vi "ReadAndConvertFile.vi"(8 "error in (no error)":errorcluster, 10 "Path":path, 11 "GXML in":refnum<class "GXML.lvclass">) -> (0 "error out":errorcluster, 2 "EPT Pattern":T1, 3 "GXML out":refnum<class "GXML.lvclass">)   [LabVIEW 2017, in "File Formats.lvlib" / "GXML.lvclass"]
uses:
  GXML.lvclass
  Parent/EST Pattern.ctl
  <vilib>/NI/GXML/_subVIs/GXML Quick Parser/Quick Parser.vi
  <vilib>/NI/GXML/GXML.lvlib
  Parent/FileFormat.lvclass
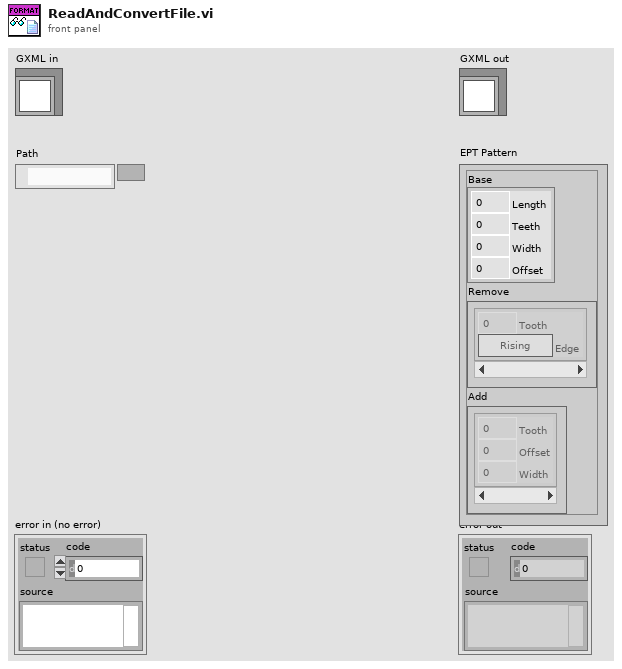
[diagram p1: front panel]
types:
  T1 = typedef "File Formats.lvlib/FileFormat.lvclass/EST Pattern.ctl" = cluster{"Base":cluster{"Length":dbl, "Teeth":u16, "Width":dbl, "Offset":dbl}, "Remove":cluster{"Tooth":u16, "Edge":bool}[], "Add":cluster{"Tooth":u16, "Offset":dbl, "Width":dbl}[]}
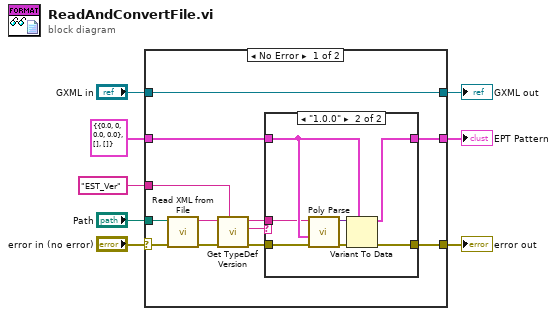
[diagram p0: block diagram]
diagram:
  n1 = case shown="No Error" "error in (no error)" {
    selector: "error in (no error)" -> [w11 w32]
    tunnel: [w12 w32] -> w8
    tunnel: [w20 w31] -> w2
    tunnel: "GXML in" -> [w20 w31]
    tunnel: "EST_Ver" -> [w14 _]
    tunnel: [w13 w30] -> w7
    tunnel: T1 {"Base"={"Length"=0.0, "Teeth"=0, "Width"=0.0, "Offset"=0.0}, "Remove"=[], "Add"=[]} ("EPT Pattern") -> [w10 w30]
    tunnel: "Path" -> [w9 _]
    frame No Error {
      n2 = call <vilib>:"Read XML from File.vi"("error in"=w11, "XML File Path"=w9) -> ("error out"=w15:errorcluster, "XML String Out"=w17:string)  [unwired: 8 in]
      n3 = call <vilib>:"Get TypeDef Version.vi"("Version Tag Name"=w14, "error in"=w15, "XML String In"=w17) -> ("error out"=w16:errorcluster, "Version String"=w19:string, "XML String Out"=w18:string)  [unwired: 6 in]
      n4 = case shown="\"1.0.0\"" w19 {
        tunnel: w10 -> [w21 w27]
        tunnel: [w21 w26] -> w13
        tunnel: [w22 w25] -> w12
        tunnel: w16 -> [w22 w24]
        tunnel: w18 -> [_ w23]
        frame Default {
        }
        frame "1.0.0" {
          n5 = call-poly <vilib>:"Poly Parse.vi"("error in"=w24, "TypeDesc"=w27, "XML File String"=w23) -> ("error out"=w29:errorcluster, "Parsed Data"=w28:variant)  [unwired: 7 in]
          n6 = Variant To Data(error in=w29, type=w27, Variant=w28) -> (data=w26:T1, error out=w25:errorcluster)
        }
      }
    }
    frame Error {
    }
  }
  "error out" <- w8
  "GXML out" <- w2
  "EPT Pattern" <- w7
